vi "Static Write.vi"(8 "error in (no error)":errorcluster, 10 "Value":ext, 11 "Abs_Extended Float in":refnum<class "Abs_Extended Float.lvclass">) -> (0 "error out":errorcluster, 3 "Abs_Extended Float out":refnum<class "Abs_Extended Float.lvclass">)   [LabVIEW 2021, in "Abs_Extended Float.lvclass"]
uses:
  Abs_Extended Float.lvclass
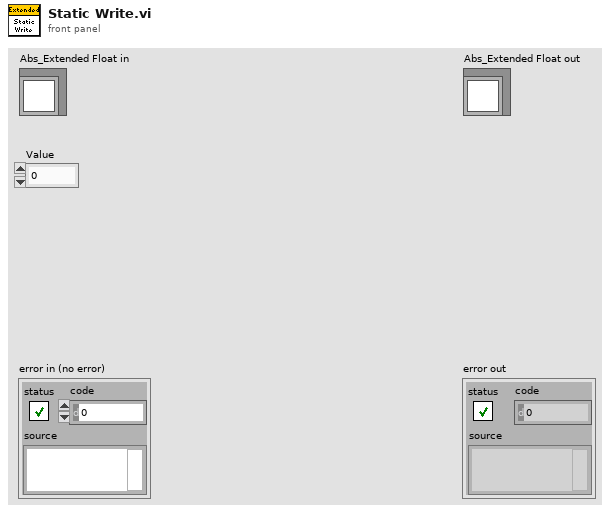
[diagram p1: front panel]
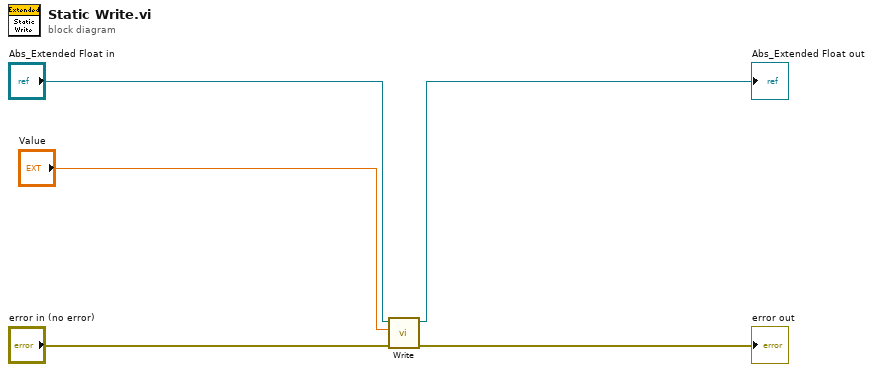
[diagram p0: block diagram]
diagram:
  n1 = call-dynamic "Write.vi"("error in (no error)"="error in (no error)", "Value"="Value", "Double Float.lvclass_340760 in"="Abs_Extended Float in") -> ("error out"=→"error out":errorcluster, "Double Float.lvclass_340760 out"=→"Abs_Extended Float out":refnum<class "Abs_Extended Float.lvclass">)  [unwired: 7 in]
